vi "pmu_Window Width Configuration.vi"(8 "error in (no error)":errorcluster, 9 "reporting rate":i16, 10 "nominal frequency":enum16{"50 Hz", "60 Hz"}(ring), 11 "Performance Class":enum8{"M Class", "P Class"}(ring)) -> (0 "error out":errorcluster, 1 "dynamic response factors":T1, 2 "frequency window width":i32, 3 "ROCOF window width":i32)   [LabVIEW 2013, in "NI_EP_PMU.lvlib"]
uses:
  <vilib>/addons/Electrical Power/PMU/NI_EP_PMU.lvlib
  <vilib>/addons/Electrical Power/PMU/Common/Controls/pmu_CFG-3 Dynamic Response Factors.ctl
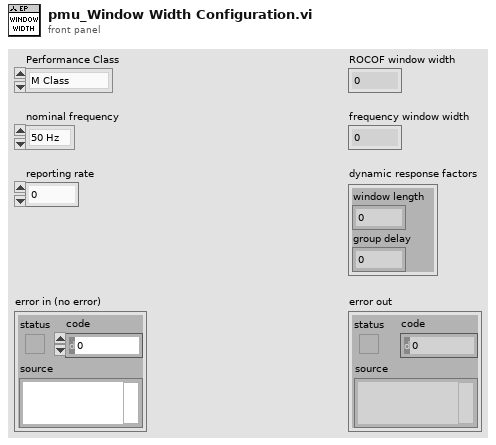
[diagram p1: front panel]
types:
  T1 = typedef "NI_EP_PMU.lvlib/pmu_CFG-3 Dynamic Response Factors.ctl" = cluster{"window length":i32, "group delay":i32}
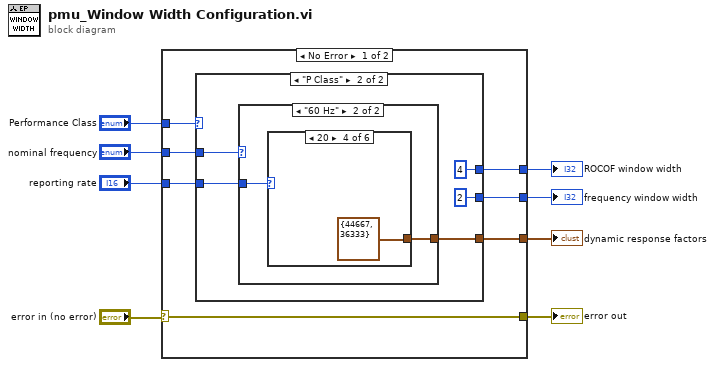
[diagram p0: block diagram]
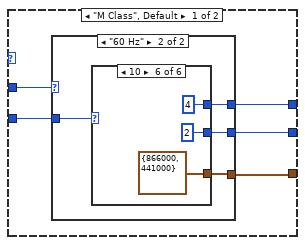
[diagram p2: hidden frame]
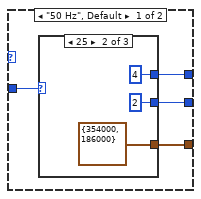
[diagram p3: hidden frame]
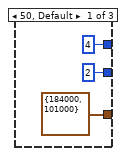
[diagram p4: hidden frame]
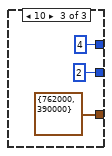
[diagram p5: hidden frame]
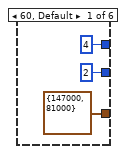
[diagram p6: hidden frame]
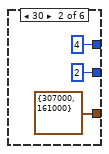
[diagram p7: hidden frame]
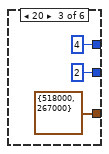
[diagram p8: hidden frame]
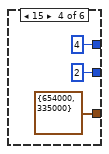
[diagram p9: hidden frame]
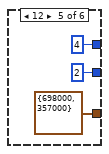
[diagram p10: hidden frame]
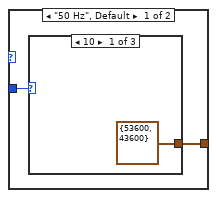
[diagram p11: hidden frame]
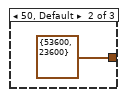
[diagram p12: hidden frame]
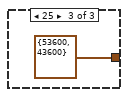
[diagram p13: hidden frame]
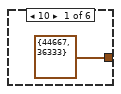
[diagram p14: hidden frame]
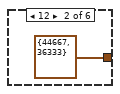
[diagram p15: hidden frame]
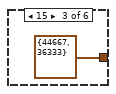
[diagram p16: hidden frame]
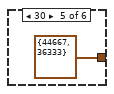
[diagram p17: hidden frame]
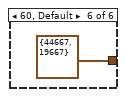
[diagram p18: hidden frame]
diagram:
  n1 = case shown="No Error" "error in (no error)" {
    selector: "error in (no error)" -> [w9 w74]
    tunnel: [w15 _] -> w8
    tunnel: "Performance Class" -> [w14 _]
    tunnel: "reporting rate" -> [w13 _]
    tunnel: "nominal frequency" -> [w12 _]
    tunnel: [w11 _] -> w4
    tunnel: [w10 _] -> w3
    tunnel: [w9 w74] -> w1
    frame No Error {
      n2 = case shown="\"P Class\"" w14 {
        tunnel: [w20 4 ("window width")] -> w11
        tunnel: w12 -> [w19 w58]
        tunnel: w13 -> [w18 w57]
        tunnel: [w17 2 ("window width")] -> w15
        tunnel: [w16 w56] -> w10
        frame "M Class", Default {
          n3 = case shown="\"60 Hz\"" w19 {
            tunnel: w18 -> [w24 w37]
            tunnel: [w23 w36] -> w20
            tunnel: [w22 w35] -> w17
            tunnel: [w21 w34] -> w16
            frame "50 Hz", Default {
              n4 = case shown="25" w24 {
                tunnel: [4 ("window width") 4 ("window width") 4 ("window width")] -> w23
                tunnel: [2 ("window width") 2 ("window width") 2 ("window width")] -> w22
                tunnel: [T1 {"window length"=184000, "group delay"=101000} ("window and group delay") T1 {"window length"=354000, "group delay"=186000} ("window and group delay") T1 {"window length"=762000, "group delay"=390000} ("window and group delay")] -> w21
                frame 50, Default {
                }
                frame 25 {
                }
                frame 10 {
                }
              }
            }
            frame "60 Hz" {
              n5 = case shown="10" w37 {
                tunnel: [4 ("window width") 4 ("window width") 4 ("window width") 4 ("window width") 4 ("window width") 4 ("window width")] -> w36
                tunnel: [2 ("window width") 2 ("window width") 2 ("window width") 2 ("window width") 2 ("window width") 2 ("window width")] -> w35
                tunnel: [T1 {"window length"=147000, "group delay"=81000} ("window and group delay") T1 {"window length"=307000, "group delay"=161000} ("window and group delay") T1 {"window length"=518000, "group delay"=267000} ("window and group delay") T1 {"window length"=654000, "group delay"=335000} ("window and group delay") T1 {"window length"=698000, "group delay"=357000} ("window and group delay") T1 {"window length"=866000, "group delay"=441000} ("window and group delay")] -> w34
                frame 60, Default {
                }
                frame 30 {
                }
                frame 20 {
                }
                frame 15 {
                }
                frame 12 {
                }
                frame 10 {
                }
              }
            }
          }
        }
        frame "P Class" {
          n6 = case shown="\"60 Hz\"" w58 {
            tunnel: w57 -> [w62 w67]
            tunnel: [w61 w66] -> w56
            frame "50 Hz", Default {
              n7 = case shown="10" w62 {
                tunnel: [T1 {"window length"=53600, "group delay"=43600} ("window and group delay") T1 {"window length"=53600, "group delay"=23600} ("window and group delay") T1 {"window length"=53600, "group delay"=43600} ("window and group delay")] -> w61
                frame 10 {
                }
                frame 50, Default {
                }
                frame 25 {
                }
              }
            }
            frame "60 Hz" {
              n8 = case shown="20" w67 {
                tunnel: [T1 {"window length"=44667, "group delay"=36333} ("window and group delay") T1 {"window length"=44667, "group delay"=36333} ("window and group delay") T1 {"window length"=44667, "group delay"=36333} ("window and group delay") T1 {"window length"=44667, "group delay"=36333} ("window and group delay") T1 {"window length"=44667, "group delay"=36333} ("window and group delay") T1 {"window length"=44667, "group delay"=19667} ("window and group delay")] -> w66
                frame 10 {
                }
                frame 12 {
                }
                frame 15 {
                }
                frame 20 {
                }
                frame 30 {
                }
                frame 60, Default {
                }
              }
            }
          }
        }
      }
    }
    frame Error {
    }
  }
  "frequency window width" <- w8
  "ROCOF window width" <- w4
  "dynamic response factors" <- w3
  "error out" <- w1
